vi "Step down array.vi"(8 "Steps":u16=5, 9 "Sorted":bool, 10 "Range":dbl=1.0, 11 "Center":dbl) -> (3 "Array":dbl[](graph)=[0.0, -0.25, 0.25, -0.5, 0.5])   [LabVIEW 2018]
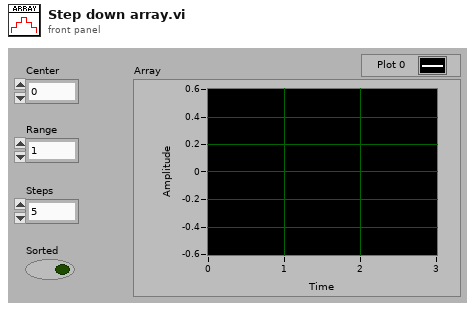
[diagram p1: front panel]
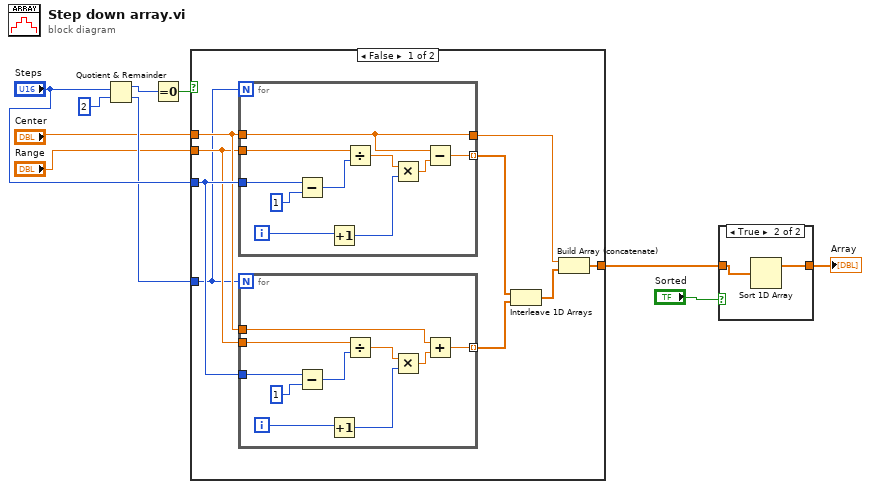
[diagram p0: block diagram]
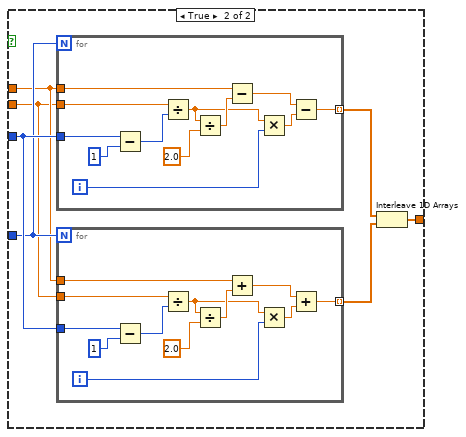
[diagram p3: hidden frame]
diagram:
  n1 = Quotient & Remainder(x="Steps", y=u16 2) -> (x-y*floor(x/y)=w9:u16, floor(x/y)=w7:u16)
  n2 = Equal To 0?(x=w9) -> (x = 0?=w6:bool)
  n3 = case shown="False" w6 {
    tunnel: "Steps" -> [w17 w46]
    tunnel: w7 -> [w11 w45]
    tunnel: [w14 w42] -> w3
    tunnel: "Center" -> [w13 w41]
    tunnel: "Range" -> [w12 w40]
    frame False {
      n4 = for {
        N: w11 -> [_]
        tunnel: [w25] -> w19 mode=indexing
        tunnel: w17 -> [w23]
        tunnel: [w21] -> w15
        tunnel: w13 -> [w21]
        tunnel: w12 -> [w20]
        i -> [w24]
        n5 = Subtract(x=w23, y=u16 1) -> (x-y=w28:u16)
        n6 = Increment(x=w24) -> (x+1=w22:i32)
        n7 = Divide(x=w20, y=w28) -> (x/y=w27:dbl)
        n8 = Multiply(x=w27, y=w22) -> (x*y=w26:dbl)
        n9 = Subtract(x=w21, y=w26) -> (x-y=w25:dbl)
      }
      n10 = for {
        N: w11 -> [_]
        tunnel: [w35] -> w18 mode=indexing
        tunnel: w17 -> [w33]
        tunnel: w13 -> [w31]
        tunnel: w12 -> [w30]
        i -> [w34]
        n11 = Subtract(x=w33, y=u16 1) -> (x-y=w38:u16)
        n12 = Increment(x=w34) -> (x+1=w32:i32)
        n13 = Divide(x=w30, y=w38) -> (x/y=w37:dbl)
        n14 = Multiply(x=w37, y=w32) -> (x*y=w36:dbl)
        n15 = Add(x=w31, y=w36) -> (x+y=w35:dbl)
      }
      n16 = Interleave 1D Arrays(w19, w18) -> (w16:dbl[])
      n17 = Build Array (concatenate)(w15, w16) -> (w14:dbl[])
    }
    frame True {
      n18 = for {
        N: w45 -> [_]
        tunnel: w46 -> [w70]
        tunnel: [w62] -> w44 mode=indexing
        tunnel: w41 -> [w60]
        tunnel: w40 -> [w59]
        i -> [w61]
        n19 = Subtract(x=w70, y=u16 1) -> (x-y=w68:u16)
        n20 = Divide(x=w59, y=w68) -> (x/y=w65:dbl)
        n21 = Divide(x=w65, y=2.0) -> (x/y=w66:dbl)
        n22 = Subtract(x=w60, y=w66) -> (x-y=w63:dbl)
        n23 = Multiply(x=w65, y=w61) -> (x*y=w64:dbl)
        n24 = Subtract(x=w63, y=w64) -> (x-y=w62:dbl)
      }
      n25 = for {
        N: w45 -> [_]
        tunnel: [w51] -> w43 mode=indexing
        tunnel: w46 -> [w49]
        tunnel: w41 -> [w48]
        tunnel: w40 -> [w47]
        i -> [w50]
        n26 = Subtract(x=w49, y=u16 1) -> (x-y=w57:u16)
        n27 = Divide(x=w47, y=w57) -> (x/y=w54:dbl)
        n28 = Divide(x=w54, y=2.0) -> (x/y=w55:dbl)
        n29 = Add(x=w48, y=w55) -> (x+y=w52:dbl)
        n30 = Multiply(x=w54, y=w50) -> (x*y=w53:dbl)
        n31 = Add(x=w52, y=w53) -> (x+y=w51:dbl)
      }
      n32 = Interleave 1D Arrays(w44, w43) -> (w42:dbl[])
    }
  }
  n33 = case shown="True" "Sorted" {
    tunnel: w3 -> [w71 w73]
    tunnel: [w71 w72] -> w2
    frame False {
    }
    frame True {
      n34 = Sort 1D Array(array=w73) -> (sorted array=w72:dbl[])
    }
  }
  "Array" <- w2
